vi "Remove dB.vi"(10 "View":T1, 11 "Average FRF in":cluster{"x0":dbl, "df":dbl, dbl[]}) -> (3 "Average FRF out":cluster{"x0":dbl, "df":dbl, dbl[]})   [LabVIEW 2022 SP3]
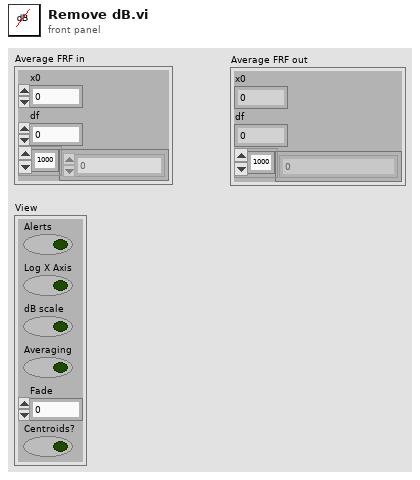
[diagram p1: front panel]
types:
  T1 = cluster{"Alerts":bool, "Log X Axis":bool, "dB scale":bool, "Averaging":bool, "Fade":dbl, "Centroids?":bool}
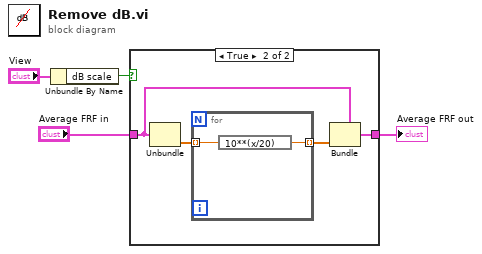
[diagram p0: block diagram]
diagram:
  n1 = Unbundle By Name("View") -> ("dB scale"=w4:bool)
  n2 = case shown="True" w4 {
    tunnel: "Average FRF in" -> [w5 w7]
    tunnel: [w5 w6] -> w3
    frame False {
    }
    frame True {
      n3 = Unbundle(w7) -> (w9:dbl[])  [unwired: 2 out]
      n4 = for {
        tunnel: w9 -> [w11] mode=indexing
        tunnel: [w10] -> w8 mode=indexing
        n5 = expression code="10**(x/20)"(w11) -> (w10:dbl)
      }
      n6 = Bundle(cluster=w7, w8) -> (w6:cluster{"x0":dbl, "df":dbl, dbl[]})  [unwired: 2 in]
    }
  }
  "Average FRF out" <- w3
